vi "USB通讯实验.vi"() -> ()   [LabVIEW 2011]
uses:
  <vilib>/STM32_DriverVI_Interface_F4/USB/USB Connect_F4.ctl
  <vilib>/STM32_DriverVI_Interface_F4/USB/USB EPX OUT_F4.ctl
  <vilib>/STM32_DriverVI_Interface_F4/USB/USB EPX IN_F4.ctl
  <vilib>/STM32_DriverVI_Interface_F4/USB/USB Read Data_Str_F4.vi
  <vilib>/STM32_DriverVI_Interface_F4/USB/USB Send Data_Str_F4.vi
panel:
  out "数值":i32
  out "USB Read Data":string="dlw30@126.com"
  in  "Data_Bytes（MAX:1024）":u16=64
  out "Init_Success?":bool
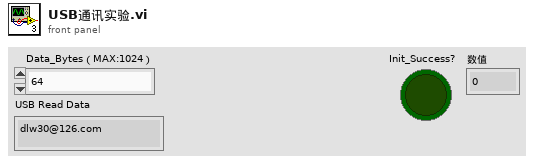
[diagram p1: front panel]
types:
  T1 = typedef "USB Connect_F4.ctl" = enum8{"Disconnect", "Connected"}
  T2 = typedef "USB EPX OUT_F4.ctl" = u8
  T3 = typedef "USB EPX IN_F4.ctl" = u8
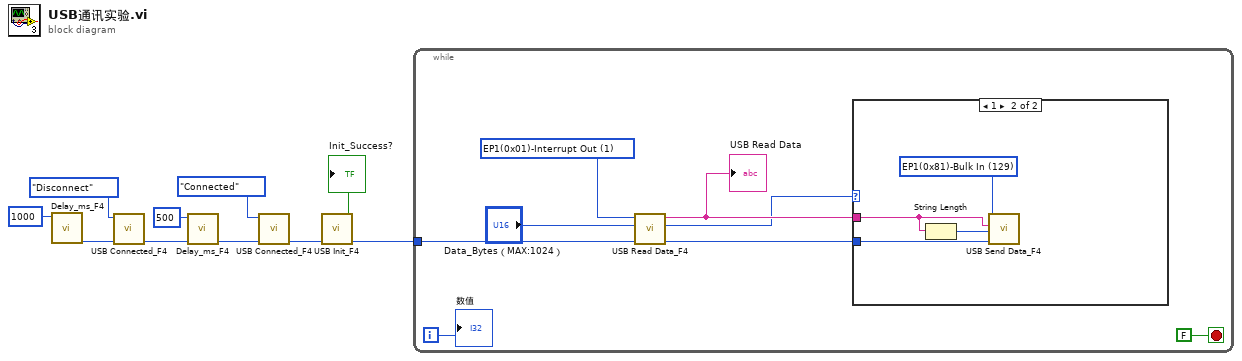
[diagram p0: block diagram]
diagram:
  n1 = call <vilib>:"Delay_ms_F4.vi"("time_ms"=u32 1000) -> ("err_out"=w9:u8)  [unwired: 10 in]
  n2 = call <vilib>:"USB Connected_F4.vi"("err_in"=w9, "USB Connect_Disconnect"=USB_Connect_F4."Disconnect") -> ("err_out"=w7:u8)  [unwired: 9 in]
  n3 = call <vilib>:"Delay_ms_F4.vi"("err_in"=w7, "time_ms"=u32 500) -> ("err_out"=w5:u8)  [unwired: 9 in]
  n4 = call <vilib>:"USB Connected_F4.vi"("err_in"=w5, "USB Connect_Disconnect"=USB_Connect_F4."Connected") -> ("err_out"=w3:u8)  [unwired: 9 in]
  n5 = call <vilib>:"USB Init_F4.vi"("err_in"=w3) -> ("err_out"=w1:u8, "Init_Success?"=→"Init_Success?":bool)  [unwired: 9 in]
  n6 = while {
    tunnel: w1 -> [w18]
    i -> [w11]
    stop <- FALSE stop-if-true
    w17 = T2 1 items=["EP1(0x01)-Interrupt Out"=1] ("USB EP_X Out Type")
    n7 = call-poly <vilib>:"USB Read Data_F4.vi"("err_in"=w18, "Data_Bytes（MAX:1024）"="Data_Bytes（MAX:1024）", "USB EP_X Out Type"=w17) -> ("err_out"=w15:u8, "Read_Num"=w13:u16, "USB Read Data"=w14:string)  [unwired: 6 in]
    "USB Read Data" <- w14
    n8 = case shown="1" w13 {
      tunnel: w15 -> [_ w22]
      tunnel: w14 -> [_ w19]
      frame 0, Default {
      }
      frame 1 {
        w21 = T3 129 items=["EP1(0x81)-Bulk In"=129] ("USB EP_X In Type")
        n9 = String Length(string=w19) -> (length=w20:i32)
        n10 = call-poly <vilib>:"USB Send Data_F4.vi"("err_in"=w22, "Data_Bytes（MAX:64）"=w20, "USB Write Data"=w19, "USB EP_X In Type"=w21) -> ()  [unwired: 6 in, 2 out]
      }
    }
    "数值" <- w11
  }
